vi "rsscope_core_global.vi"() -> ()   [LabVIEW 2014] (continued)
"Access"=2, "Range Table"="RsScope_rngPowerQualityCustomFrequency", "Read Callback"="", "Write Callback"="", "Supported Models"="", "Instrument Options"="", "Flags"=0, "Help"="Sets the user-defined frequency if RSSCOPE_ATTR_POWER_QUALITY_FREQUENCY is set to Custom.\n\nAvailable Repeated Capabilities:\nNone\n\nRemote-control command(s):\nPOWer:QUALity:FCUS"}, {"Level"=3, "Class Only"=FALSE, "Identifier"="RSSCOPE_ATTR_POWER_QUALITY_SCALING", "Descriptive Name"="Power Quality Scaling", "Data Type"=0, "Command"="POW:QUAL:AUTO", "Access"=2, "Range Table"="RsScope_rngPowerScaling", "Read Callback"="", "Write Callback"="", "Supported Models"="", "Instrument Options"="", "Flags"=0, "Help"="Selects the scaling for the display of the results.\n\nAvailable Repeated Capabilities:\nNone\n\nRemote-control command(s):\nPOWer:QUALity:AUTO"}, {"Level"=3, "Class Only"=FALSE, "Identifier"="RSSCOPE_ATTR_POWER_QUALITY_ADD", "Descriptive Name"="Power Quality Add To Report", "Data Type"=4, "Command"="POW:QUAL:REP:ADD", "Access"=1, "Range Table"="", "Read Callback"="", "Write Callback"="", "Supported Models"="", "Instrument Options"="", "Flags"=0, "Help"="Adds the result to the report list.\n\nAvailable Repeated Capabilities:\nNone\n\nRemote-control command(s):\nPOWer:QUALity:REPort:ADD"}, {"Level"=3, "Class Only"=TRUE, "Identifier"="", "Descriptive Name"="Results", "Data Type"=0, "Command"="", "Access"=0, "Range Table"="", "Read Callback"="", "Write Callback"="", "Supported Models"="", "Instrument Options"="", "Flags"=0, "Help"="Power quality measurement results."}, {"Level"=2, "Class Only"=TRUE, "Identifier"="", "Descriptive Name"="Current Harmonics", "Data Type"=0, "Command"="", "Access"=0, "Range Table"="", "Read Callback"="", "Write Callback"="", "Supported Models"="", "Instrument Options"="", "Flags"=0, "Help"="Current Harmonics"}, {"Level"=3, "Class Only"=FALSE, "Identifier"="RSSCOPE_ATTR_START_POWER_CURRENT_HARMONICS", "Descriptive Name"="Start Power Current Harmonics Measurement", "Data Type"=4, "Command"="POW:HARM:EXEC", "Access"=1, "Range Table"="", "Read Callback"="", "Write Callback"="", "Supported Models"="", "Instrument Options"="", "Flags"=0, "Help"="Start power current harmonics measurement.\n\nAvailable Repeated Capabilities:\nNone\n\nRemote-control command(s):\nPOWer:HARMonics:EXECute"}, {"Level"=3, "Class Only"=FALSE, "Identifier"="RSSCOPE_ATTR_POWER_CURRENT_HARMONICS_STANDARD", "Descriptive Name"="Power Current Harmonics Standard", "Data Type"=0, "Command"="POW:HARM:STAN", "Access"=2, "Range Table"="RsScope_rngPowerCurrentHarmonicsStandard", "Read Callback"="", "Write Callback"="", "Supported Models"="", "Instrument Options"="", "Flags"=0, "Help"="Selects current harmonics standard.\n\nAvailable Repeated Capabilities:\nNone\n\nRemote-control command(s):\nPOWer:HARMonics:STAN"}, {"Level"=3, "Class Only"=FALSE, "Identifier"="RSSCOPE_ATTR_POWER_CURRENT_HARMONICS_EN_FREQUENCY", "Descriptive Name"="Power Current Harmonics EN Frequency", "Data Type"=0, "Command"="POW:HARM:ENFR", "Access"=2, "Range Table"="RsScope_rngPowerCurrentHarmonicsFrequency", "Read Callback"="", "Write Callback"="", "Supported Models"="", "Instrument Options"="", "Flags"=0, "Help"="Selects the frequency of the input signal for the EN 61000-3-2 Class standards.\nValues F_50 and F_60 are valid for this command.\n\nAvailable Repeated Capabilities:\nNone\n\nRemote-control command(s):\nPOWer:HARMonics:ENFR"}, {"Level"=3, "Class Only"=FALSE, "Identifier"="RSSCOPE_ATTR_POWER_CURRENT_HARMONICS_MI_FREQUENCY", "Descriptive Name"="Power Current Harmonics MI Frequency", "Data Type"=0, "Command"="POW:HARM:MIFR", "Access"=2, "Range Table"="RsScope_rngPowerCurrentHarmonicsFrequency", "Read Callback"="", "Write Callback"="", "Supported Models"="", "Instrument Options"="", "Flags"=0, "Help"="Selects the frequency of the input signal for the MIL-STD-1399 standard.\nF_60 and F_400 are valid for this command\n\nAvailable Repeated Capabilities:\nNone\n\nRemote-control command(s):\nPOWer:HARMonics:MIFR"}, {"Level"=3, "Class Only"=FALSE, "Identifier"="RSSCOPE_ATTR_POWER_CURRENT_HARMONICS_DO_FREQUENCY", "Descriptive Name"="Power Current Harmonics DO Frequency", "Data Type"=0, "Command"="POW:HARM:DOFR", "Access"=2, "Range Table"="RsScope_rngPowerCurrentHarmonicsFrequency", "Read Callback"="", "Write Callback"="", "Supported Models"="", "Instrument Options"="", "Flags"=0, "Help"="Selects the frequency of the input signal for theRTCA DO-160 standard.\nValues F_360, F_400, F_650, F_800 are valid for this command\n\nAvailable Repeated Capabilities:\nNone\n\nRemote-control command(s):\nPOWer:HARMonics:DOFR"}, {"Level"=3, "Class Only"=FALSE, "Identifier"="RSSCOPE_ATTR_POWER_CURRENT_HARMONICS_EVALUATION", "Descriptive Name"="Power Current Harmonics Evaluation", "Data Type"=0, "Command"="POW:HARM:EVAL", "Access"=2, "Range Table"="RsScope_rngPowerCurrentHarmonicsEvaluation", "Read Callback"="", "Write Callback"="", "Supported Models"="", "Instrument Options"="", "Flags"=0, "Help"="Selects how the results are evaluated.\n\nAvailable Repeated Capabilities:\nNone\n\nRemote-control command(s):\nPOWer:HARMonics:EVAL"}, {"Level"=3, "Class Only"=FALSE, "Identifier"="RSSCOPE_ATTR_POWER_CURRENT_HARMONICS_EVALUATION_VOLT", "Descriptive Name"="Power Current Harmonics Evaluation Voltage", "Data Type"=0, "Command"="POW:HARM:VOLT", "Access"=2, "Range Table"="RsScope_rngPowerCurrentHarmonicsVoltageResultsDisplay", "Read Callback"="", "Write Callback"="", "Supported Models"="", "Instrument Options"="", "Flags"=0, "Help"="Selects if the voltage results are displayed or not for &apos;Standard&apos; > &apos;RTCA DO-160&apos; and enabled &apos;Evaluation with voltage source and revised current law&apos;.\n\nAvailable Repeated Capabilities:\nNone\n\nRemote-control command(s):\nPOWer:HARMonics:VOLT"}, {"Level"=3, "Class Only"=FALSE, "Identifier"="RSSCOPE_ATTR_POWER_CURRENT_HARMONICS_SCALING", "Descriptive Name"="Power Current Harmonics Scaling", "Data Type"=0, "Command"="POW:HARM:AUTO", "Access"=2, "Range Table"="RsScope_rngPowerScaling", "Read Callback"="", "Write Callback"="", "Supported Models"="", "Instrument Options"="", "Flags"=0, "Help"="Selects the scaling for the display of the results.\n\nAvailable Repeated Capabilities:\nNone\n\nRemote-control command(s):\nPOWer:HARMonics:AUTO"}, {"Level"=3, "Class Only"=FALSE, "Identifier"="RSSCOPE_ATTR_POWER_CURRENT_HARMONICS_ADD", "Descriptive Name"="Power Current Harmonics Add To Report", "Data Type"=4, "Command"="POW:HARM:REP:ADD", "Access"=1, "Range Table"="", "Read Callback"="", "Write Callback"="", "Supported Models"="", "Instrument Options"="", "Flags"=0, "Help"="Adds the result to the report list.\n\nAvailable Repeated Capabilities:\nNone\n\nRemote-control command(s):\nPOWer:HARMonics:REPort:ADD"}, {"Level"=3, "Class Only"=TRUE, "Identifier"="", "Descriptive Name"="Results", "Data Type"=0, "Command"="", "Access"=0, "Range Table"="", "Read Callback"="", "Write Callback"="", "Supported Models"="", "Instrument Options"="", "Flags"=0, "Help"="Current harmonics measurement results."}, {"Level"=4, "Class Only"=FALSE, "Identifier"="RSSCOPE_ATTR_POWER_CURRENT_HARMONICS_USED_STANDARD", "Descriptive Name"="Power Current Harmonics Used Standard", "Data Type"=0, "Command"="POW:HARM:RES{ResultNumber}:STD?", "Access"=0, "Range Table"="RsScope_rngPowerCurrentHarmonicsStandard", "Read Callback"="", "Write Callback"="", "Supported Models"="", "Instrument Options"="", "Flags"=0, "Help"="Returns the used standard.\n\nAvailable Repeated Capabilities:\nResultNumber: Res1, Res2, Res3, Res4, Res5, Res6, Res7, Res8\r\n\nRemote-control command(s):\nPOWer:HARMonics:RESult<m>:STDinuse?"}, {"Level"=4, "Class Only"=TRUE, "Identifier"="", "Descriptive Name"="Harmonic", "Data Type"=0, "Command"="", "Access"=0, "Range Table"="", "Read Callback"="", "Write Callback"="", "Supported Models"="", "Instrument Options"="", "Flags"=0, "Help"="Functions with repeated capabilty ResultHarmonics"}, {"Level"=5, "Class Only"=FALSE, "Identifier"="RSSCOPE_ATTR_POWER_CURRENT_HARMONICS_RESULT_FREQUENCY", "Descriptive Name"="Power Current Harmonics Result Frequency", "Data Type"=1, "Command"="POW:HARM:RES{ResultNumber}:FREQ{ResultHarmonics}:VAL?", "Access"=0, "Range Table"="", "Read Callback"="", "Write Callback"="", "Supported Models"="", "Instrument Options"="", "Flags"=0, "Help"="Returns the frequency for selected result and harmonic.\n\nAvailable Repeated Capabilities:\nResultNumber: Res1, Res2, Res3, Res4, Res5, Res6, Res7, Res8\r\nResultHarmonics: Harm1, Harm2, Harm3, Harm4, Harm5, Harm6, Harm7, Harm8, Harm9, Harm10, Harm11, Harm12, Harm13, Harm14, Harm15, Harm16, Harm17, Harm18, Harm19, Harm20, Harm21, Harm22, Harm23, Harm24, Harm25, Harm26, Harm27, Harm28, Harm29, Harm30, Harm31, Harm32, Harm33, Harm34, Harm35, Harm36, Harm37, Harm38, Harm39, Herm40\r\n\nRemote-control command(s):\nPOWer:HARMonics:RESult<m>:FREQuency<n>:VALue?"}, {"Level"=5, "Class Only"=FALSE, "Identifier"="RSSCOPE_ATTR_POWER_CURRENT_HARMONICS_RESULT_MAX", "Descriptive Name"="Power Current Harmonics Result Maximum", "Data Type"=1, "Command"="POW:HARM:RES{ResultNumber}:MAXV{ResultHarmonics}:VAL?", "Access"=0, "Range Table"="", "Read Callback"="", "Write Callback"="", "Supported Models"="", "Instrument Options"="", "Flags"=0, "Help"="Returns the maximum measured value for selected result and harmonic.\n\nAvailable Repeated Capabilities:\nResultNumber: Res1, Res2, Res3, Res4, Res5, Res6, Res7, Res8\r\nResultHarmonics: Harm1, Harm2, Harm3, Harm4, Harm5, Harm6, Harm7, Harm8, Harm9, Harm10, Harm11, Harm12, Harm13, Harm14, Harm15, Harm16, Harm17, Harm18, Harm19, Harm20, Harm21, Harm22, Harm23, Harm24, Harm25, Harm26, Harm27, Harm28, Harm29, Harm30, Harm31, Harm32, Harm33, Harm34, Harm35, Harm36, Harm37, Harm38, Harm39, Herm40\r\n\nRemote-control command(s):\nPOWer:HARMonics:RESult<m>:MAXValue<n>:VALue?"}, {"Level"=5, "Class Only"=FALSE, "Identifier"="RSSCOPE_ATTR_POWER_CURRENT_HARMONICS_RESULT_STD", "Descriptive Name"="Power Current Harmonics Result Standard Limit", "Data Type"=1, "Command"="POW:HARM:RES{ResultNumber}:STDV{ResultHarmonics}:VAL?", "Access"=0, "Range Table"="", "Read Callback"="", "Write Callback"="", "Supported Models"="", "Instrument Options"="", "Flags"=0, "Help"="Returns the maxim alowed value according selected standard for selected result and harmonic.\n\nAvailable Repeated Capabilities:\nResultNumber: Res1, Res2, Res3, Res4, Res5, Res6, Res7, Res8\r\nResultHarmonics: Harm1, Harm2, Harm3, Harm4, Harm5, Harm6, Harm7, Harm8, Harm9, Harm10, Harm11, Harm12, Harm13, Harm14, Harm15, Harm16, Harm17, Harm18, Harm19, Harm20, Harm21, Harm22, Harm23, Harm24, Harm25, Harm26, Harm27, Harm28, Harm29, Harm30, Harm31, Harm32, Harm33, Harm34, Harm35, Harm36, Harm37, Harm38, Harm39, Herm40\r\n\nRemote-control command(s):\nPOWer:HARMonics:RESult<m>:STDValue<n>:VALue?"}, {"Level"=5, "Class Only"=FALSE, "Identifier"="RSSCOPE_ATTR_POWER_CURRENT_HARMONICS_RESULT_VALUE", "Descriptive Name"="Power Current Harmonics Result Value", "Data Type"=1, "Command"="POW:HARM:RES{ResultNumber}:VAL{ResultHarmonics}:VAL?", "Access"=0, "Range Table"="", "Read Callback"="", "Write Callback"="", "Supported Models"="", "Instrument Options"="", "Flags"=0, "Help"="Returns the present value for selected result and harmonic.\n\nAvailable Repeated Capabilities:\nResultNumber: Res1, Res2, Res3, Res4, Res5, Res6, Res7, Res8\r\nResultHarmonics: Harm1, Harm2, Harm3, Harm4, Harm5, Harm6, Harm7, Harm8, Harm9, Harm10, Harm11, Harm12, Harm13, Harm14, Harm15, Harm16, Harm17, Harm18, Harm19, Harm20, Harm21, Harm22, Harm23, Harm24, Harm25, Harm26, Harm27, Harm28, Harm29, Harm30, Harm31, Harm32, Harm33, Harm34, Harm35, Harm36, Harm37, Harm38, Harm39, Herm40\r\n\nRemote-control command(s):\nPOWer:HARMonics:RESult<m>:VALue<n>:VALue?"}, {"Level"=2, "Class Only"=TRUE, "Identifier"="", "Descriptive Name"="Inrush Current", "Data Type"=0, "Command"="", "Access"=0, "Range Table"="", "Read Callback"="", "Write Callback"="", "Supported Models"="", "Instrument Options"="", "Flags"=0, "Help"="Inrush current measurement."}, {"Level"=3, "Class Only"=FALSE, "Identifier"="RSSCOPE_ATTR_START_POWER_INRUSH_CURRENT_MEASUREMENT", "Descriptive Name"="Start Power Inrush Current Measurement", "Data Type"=4, "Command"="POW:INR:EXEC", "Access"=1, "Range Table"="", "Read Callback"="", "Write Callback"="", "Supported Models"="", "Instrument Options"="", "Flags"=0, "Help"="Start power inrush current measurement.\n\nAvailable Repeated Capabilities:\nNone\n\nRemote-control command(s):\nPOWer:INRush:EXECute"}, {"Level"=3, "Class Only"=FALSE, "Identifier"="RSSCOPE_ATTR_POWER_INRUSH_CURRENT_MAX", "Descriptive Name"="Power Inrush Current Max Current", "Data Type"=1, "Command"="POW:INR:MAXC", "Access"=2, "Range Table"="RsScope_rngPowerInrushCurrentMaxCurrent", "Read Callback"="", "Write Callback"="", "Supported Models"="", "Instrument Options"="", "Flags"=0, "Help"="Sets the maximum expected current for the vertical scale.\n\nAvailable Repeated Capabilities:\nNone\n\nRemote-control command(s):\nPOWer:INRush:MAXCurrent"}, {"Level"=3, "Class Only"=FALSE, "Identifier"="RSSCOPE_ATTR_POWER_INRUSH_CURRENT_TRIGGER", "Descriptive Name"="Power Inrush Current Trigger", "Data Type"=1, "Command"="POW:INR:TRIG", "Access"=2, "Range Table"="RsScope_rngPowerInrushCurrentTrigger", "Read Callback"="", "Write Callback"="", "Supported Models"="", "Instrument Options"="", "Flags"=0, "Help"="Sets the current value for the trigger\n\nAvailable Repeated Capabilities:\nNone\n\nRemote-control command(s):\nPOWer:INRush:TRIGger"}, {"Level"=3, "Class Only"=FALSE, "Identifier"="RSSCOPE_ATTR_POWER_INRUSH_CURRENT_ADD", "Descriptive Name"="Power Inrush Current Add To Report", "Data Type"=4, "Command"="POW:INR:REP:ADD", "Access"=1, "Range Table"="", "Read Callback"="", "Write Callback"="", "Supported Models"="", "Instrument Options"="", "Flags"=0, "Help"="Adds the result to the report list.\n\nAvailable Repeated Capabilities:\nNone\n\nRemote-control command(s):\nPOWer:INRush:REPort:ADD"}, {"Level"=3, "Class Only"=FALSE, "Identifier"="RSSCOPE_ATTR_POWER_INRUSH_CURRENT_GATE_ADD", "Descriptive Name"="Power Inrush Current Gate Add", "Data Type"=4, "Command"="POW:INR:ADD", "Access"=1, "Range Table"="", "Read Callback"="", "Write Callback"="", "Supported Models"="", "Instrument Options"="", "Flags"=0, "Help"="Adds a gate.\n\nAvailable Repeated Capabilities:\nNone\n\nRemote-control command(s):\nPOWer:INRush:ADD"}, {"Level"=3, "Class Only"=FALSE, "Identifier"="RSSCOPE_ATTR_POWER_INRUSH_CURRENT_GATE_INS", "Descriptive Name"="Power Inrush Current Gate Insert", "Data Type"=0, "Command"="POW:INR:INS", "Access"=1, "Range Table"="", "Read Callback"="", "Write Callback"="", "Supported Models"="", "Instrument Options"="", "Flags"=0, "Help"="Inserts a gate.\n\nAvailable Repeated Capabilities:\nNone\n\nRemote-control command(s):\nPOWer:INRush:INSert"}, {"Level"=3, "Class Only"=FALSE, "Identifier"="RSSCOPE_ATTR_POWER_INRUSH_CURRENT_GATE_REMOVE", "Descriptive Name"="Power Inrush Current Gate Remove", "Data Type"=0, "Command"="POW:INR:REM", "Access"=1, "Range Table"="", "Read Callback"="", "Write Callback"="", "Supported Models"="", "Instrument Options"="", "Flags"=0, "Help"="Removes a gate.\n\nAvailable Repeated Capabilities:\nNone\n\nRemote-control command(s):\nPOWer:INRush:REMove"}, {"Level"=3, "Class Only"=FALSE, "Identifier"="RSSCOPE_ATTR_POWER_INRUSH_CURRENT_GATE_COUNT", "Descriptive Name"="Power Inrush Current Gate Count", "Data Type"=0, "Command"="POW:INR:COUN?", "Access"=0, "Range Table"="", "Read Callback"="", "Write Callback"="", "Supported Models"="", "Instrument Options"="", "Flags"=0, "Help"="Queiries the number of inrush current gates.\n\nAvailable Repeated Capabilities:\nNone\n\nRemote-control command(s):\nPOWer:INRush:COUNt?"}, {"Level"=3, "Class Only"=TRUE, "Identifier"="", "Descriptive Name"="Gate", "Data Type"=0, "Command"="", "Access"=0, "Range Table"="", "Read Callback"="", "Write Callback"="", "Supported Models"="", "Instrument Options"="", "Flags"=0, "Help"="Attributes with gate repeated capability.\n\nConfigures different gates (time periods). You can configure up to\nfive different gates. The time periods of the defined gates may overlap."}, {"Level"=4, "Class Only"=FALSE, "Identifier"="RSSCOPE_ATTR_POWER_INRUSH_CURRENT_GATE_VALUE", "Descriptive Name"="Power Inrush Current Gate Value", "Data Type"=1, "Command"="POW:INR:GATE{Gate}:VAL", "Access"=2, "Range Table"="RsScope_rngPowerInrushCurrentGateValue", "Read Callback"="", "Write Callback"="", "Supported Models"="", "Instrument Options"="", "Flags"=0, "Help"="Sets the value of the inrush current.\n\nAvailable Repeated Capabilities:\nGate: Gate1, Gate2, Gate3, Gate4, Gate5\r\n\nRemote-control command(s):\nPOWer:INRush:GATE<m>:VAlue"}, {"Level"=4, "Class Only"=FALSE, "Identifier"="RSSCOPE_ATTR_POWER_INRUSH_CURRENT_GATE_START", "Descriptive Name"="Power Inrush Current Gate Start", "Data Type"=1, "Command"="POW:INR:GATE{Gate}:STAR", "Access"=2, "Range Table"="RsScope_rngPowerInrushCurrentGateMeasTime", "Read Callback"="", "Write Callback"="", "Supported Models"="", "Instrument Options"="", "Flags"=0, "Help"="Sets the start measuring time for the selected gate.\n\nAvailable Repeated Capabilities:\nGate: Gate1, Gate2, Gate3, Gate4, Gate5\r\n\nRemote-control command(s):\nPOWer:INRush:GATE<m>:STARt"}, {"Level"=4, "Class Only"=FALSE, "Identifier"="RSSCOPE_ATTR_POWER_INRUSH_CURRENT_GATE_STOP", "Descriptive Name"="Power Inrush Current Gate Stop", "Data Type"=1, "Command"="POW:INR:GATE{Gate}:STOP", "Access"=2, "Range Table"="RsScope_rngPowerInrushCurrentGateMeasTime", "Read Callback"="", "Write Callback"="", "Supported Models"="", "Instrument Options"="", "Flags"=0, "Help"="Sets the stop measuring time for the selected gate.\n\nAvailable Repeated Capabilities:\nGate: Gate1, Gate2, Gate3, Gate4, Gate5\r\n\nRemote-control command(s):\nPOWer:INRush:GATE<m>:STOP"}, {"Level"=4, "Class Only"=FALSE, "Identifier"="RSSCOPE_ATTR_POWER_INRUSH_CURRENT_RESULT_VALUE", "Descriptive Name"="Power Inrush Current Result Value", "Data Type"=1, "Command"="POW:INR:GATE{Gate}:VAL?", "Access"=0, "Range Table"="", "Read Callback"="", "Write Callback"="", "Supported Models"="", "Instrument Options"="", "Flags"=0, "Help"="Returns the value of the inrush current.\n\nAvailable Repeated Capabilities:\nGate: Gate1, Gate2, Gate3, Gate4, Gate5\r\n\nRemote-control command(s):\nPOWer:INRush:GATE<m>:VALue?"}, {"Level"=2, "Class Only"=TRUE, "Identifier"="", "Descriptive Name"="Ripple", "Data Type"=0, "Command"="", "Access"=0, "Range Table"="", "Read Callback"="", "Write Callback"="", "Supported Models"="", "Instrument Options"="", "Flags"=0, "Help"="Measures the ripple of the device output."}, {"Level"=3, "Class Only"=FALSE, "Identifier"="RSSCOPE_ATTR_START_POWER_RIPPLE_MEASUREMENT", "Descriptive Name"="Start Power Ripple Measurement", "Data Type"=4, "Command"="POW:RIPP:EXEC", "Access"=1, "Range Table"="", "Read Callback"="", "Write Callback"="", "Supported Models"="", "Instrument Options"="", "Flags"=0, "Help"="Start power ripple measurement.\n\nAvailable Repeated Capabilities:\nNone\n\nRemote-control command(s):\nPOWer:RIPPle:EXECute"}, {"Level"=3, "Class Only"=FALSE, "Identifier"="RSSCOPE_ATTR_POWER_RIPPLE_CURRENT_ENABLED", "Descriptive Name"="Power Ripple Current Enabled", "Data Type"=3, "Command"="POW:RIPP:CURR", "Access"=2, "Range Table"="", "Read Callback"="", "Write Callback"="", "Supported Models"="", "Instrument Options"="", "Flags"=0, "Help"="Activates or deactivates the input current.\n\nAvailable Repeated Capabilities:\nNone\n\nRemote-control command(s):\nPOWer:RIPPle:CURRent"}, {"Level"=3, "Class Only"=FALSE, "Identifier"="RSSCOPE_ATTR_POWER_RIPPLE_FREQUENCY", "Descriptive Name"="Power Ripple Frequency", "Data Type"=1, "Command"="POW:RIPP:FREQ", "Access"=2, "Range Table"="RsScope_rngPowerSwitchingFrequency", "Read Callback"="", "Write Callback"="", "Supported Models"="", "Instrument Options"="", "Flags"=0, "Help"="Sets the SMPS switching frequency.\n\nAvailable Repeated Capabilities:\nNone\n\nRemote-control command(s):\nPOWer:RIPPle:FREQuency"}, {"Level"=3, "Class Only"=FALSE, "Identifier"="RSSCOPE_ATTR_POWER_RIPPLE_SCALING", "Descriptive Name"="Power Ripple Scaling", "Data Type"=0, "Command"="POW:RIPP:AUT", "Access"=2, "Range Table"="RsScope_rngPowerScaling", "Read Callback"="", "Write Callback"="", "Supported Models"="", "Instrument Options"="", "Flags"=0, "Help"="Selects the scaling for the display of the results.\n\nAvailable Repeated Capabilities:\nNone\n\nRemote-control command(s):\nPOWer:RIPPle:AUToscale"}, {"Level"=3, "Class Only"=FALSE, "Identifier"="RSSCOPE_ATTR_POWER_RIPPLE_ADD", "Descriptive Name"="Power Ripple Add To Report", "Data Type"=4, "Command"="POW:RIPP:REP:ADD", "Access"=1, "Range Table"="", "Read Callback"="", "Write Callback"="", "Supported Models"="", "Instrument Options"="", "Flags"=0, "Help"="Adds the result to the report list.\n\nAvailable Repeated Capabilities:\nNone\n\nRemote-control command(s):\nPOWer:RIPPle:REPort:ADD"}, {"Level"=3, "Class Only"=TRUE, "Identifier"="", "Descriptive Name"="Results", "Data Type"=0, "Command"="", "Access"=0, "Range Table"="", "Read Callback"="", "Write Callback"="", "Supported Models"="", "Instrument Options"="", "Flags"=0, "Help"="Results of the ripple analysis."}, {"Level"=2, "Class Only"=TRUE, "Identifier"="", "Descriptive Name"="Spectrum", "Data Type"=0, "Command"="", "Access"=0, "Range Table"="", "Read Callback"="", "Write Callback"="", "Supported Models"="", "Instrument Options"="", "Flags"=0, "Help"="Power spectrum measurement."}, {"Level"=3, "Class Only"=FALSE, "Identifier"="RSSCOPE_ATTR_START_POWER_SPECTRUM_MEASUREMENT", "Descriptive Name"="Start Power Spectrum Measurement", "Data Type"=4, "Command"="POW:SPEC:EXEC", "Access"=1, "Range Table"="", "Read Callback"="", "Write Callback"="", "Supported Models"="", "Instrument Options"="", "Flags"=0, "Help"="Starts the spectrum measurement.\n\nAvailable Repeated Capabilities:\nNone\n\nRemote-control command(s):\nPOWer:SPECtrum:EXECute"}, {"Level"=3, "Class Only"=FALSE, "Identifier"="RSSCOPE_ATTR_POWER_SPECTRUM_FREQUENCY", "Descriptive Name"="Power Spectrum Frequency", "Data Type"=1, "Command"="POW:SPEC:FREQ", "Access"=2, "Range Table"="RsScope_rngPowerSwitchingFrequency", "Read Callback"="", "Write Callback"="", "Supported Models"="", "Instrument Options"="", "Flags"=0, "Help"="Sets the SMPS switching frequency.\n\nAvailable Repeated Capabilities:\nNone\n\nRemote-control command(s):\nPOWer:SPECtrum:FREQuency"}, {"Level"=3, "Class Only"=FALSE, "Identifier"="RSSCOPE_ATTR_POWER_SPECTRUM_SCALING", "Descriptive Name"="Power Spectrum Scaling", "Data Type"=0, "Command"="POW:SPEC:AUT", "Access"=2, "Range Table"="RsScope_rngPowerScaling", "Read Callback"="", "Write Callback"="", "Supported Models"="", "Instrument Options"="", "Flags"=0, "Help"="Selects the scaling for the display of the results.\n\nAvailable Repeated Capabilities:\nNone\n\nRemote-control command(s):\nPOWer:SPECtrum:AUToscale"}, {"Level"=3, "Class Only"=FALSE, "Identifier"="RSSCOPE_ATTR_POWER_SPECTRUM_ADD", "Descriptive Name"="Power Spectrum Add To Report", "Data Type"=4, "Command"="POW:SPEC:REP:ADD", "Access"=1, "Range Table"="", "Read Callback"="", "Write Callback"="", "Supported Models"="", "Instrument Options"="", "Flags"=0, "Help"="Adds the result to the report list.\n\nAvailable Repeated Capabilities:\nNone\n\nRemote-control command(s):\nPOWer:SPECtrum:REPort:ADD"}, {"Level"=3, "Class Only"=TRUE, "Identifier"="", "Descriptive Name"="Results", "Data Type"=0, "Command"="", "Access"=0, "Range Table"="", "Read Callback"="", "Write Callback"="", "Supported Models"="", "Instrument Options"="", "Flags"=0, "Help"="Power Spectrum Measurement Results."}, {"Level"=4, "Class Only"=FALSE, "Identifier"="RSSCOPE_ATTR_POWER_SPECTRUM_MEASUREMENT_RESULT_COUNT", "Descriptive Name"="Result Count", "Data Type"=0, "Command"="POW:SPEC:RCO?", "Access"=0, "Range Table"="", "Read Callback"="", "Write Callback"="", "Supported Models"="", "Instrument Options"="", "Flags"=0, "Help"="Returns the total number of harmonics.\n\nAvailable Repeated Capabilities:\nNone\n\nRemote-control command(s):\nPOWer:SPECtrum:RCOunt?"}, {"Level"=4, "Class Only"=FALSE, "Identifier"="RSSCOPE_ATTR_POWER_SPECTRUM_MEASUREMENT_FREQUENCY_RESULT", "Descriptive Name"="Power Spectrum Measurement Frequency Result", "Data Type"=1, "Command"="POW:SPEC:RES{ResultNumber}:FREQ?", "Access"=0, "Range Table"="", "Read Callback"="", "Write Callback"="", "Supported Models"="", "Instrument Options"="", "Flags"=0, "Help"="Returns the result frequency.\n\nAvailable Repeated Capabilities:\nResultNumber: Res1, Res2, Res3, Res4, Res5, Res6, Res7, Res8\r\n\nRemote-control command(s):\nPOWer:SPECtrum:RESult<m>:FREQuency?"}, {"Level"=4, "Class Only"=FALSE, "Identifier"="RSSCOPE_ATTR_POWER_SPECTRUM_MEASUREMENT_LEVEL_RESULT", "Descriptive Name"="Power Spectrum Measurement Level Result", "Data Type"=1, "Command"="POW:SPEC:RES{ResultNumber}:LEV?", "Access"=0, "Range Table"="", "Read Callback"="", "Write Callback"="", "Supported Models"="", "Instrument Options"="", "Flags"=0, "Help"="Returns the result level.\n\nAvailable Repeated Capabilities:\nResultNumber: Res1, Res2, Res3, Res4, Res5, Res6, Res7, Res8\r\n\nRemote-control command(s):\nPOWer:SPECtrum:RESult<m>:LEVel?"}, {"Level"=2, "Class Only"=TRUE, "Identifier"="", "Descriptive Name"="Slew Rate", "Data Type"=0, "Command"="", "Access"=0, "Range Table"="", "Read Callback"="", "Write Callback"="", "Supported Models"="", "Instrument Options"="", "Flags"=0, "Help"="Slew rate measurement."}, {"Level"=3, "Class Only"=FALSE, "Identifier"="RSSCOPE_ATTR_START_POWER_SLEW_RATE_MEASUREMENT", "Descriptive Name"="Start Power Slew Rate Measurement", "Data Type"=4, "Command"="POW:SLEW:EXEC", "Access"=1, "Range Table"="", "Read Callback"="", "Write Callback"="", "Supported Models"="", "Instrument Options"="", "Flags"=0, "Help"="Starts the slew rate measurement.\n\nAvailable Repeated Capabilities:\nNone\n\nRemote-control command(s):\nPOWer:SLEWrate:EXECute"}, {"Level"=3, "Class Only"=FALSE, "Identifier"="RSSCOPE_ATTR_POWER_SLEW_RATE_SOURCE", "Descriptive Name"="Power Slew Rate Source", "Data Type"=0, "Command"="POW:SLEW:SOUR", "Access"=2, "Range Table"="RsScope_rngPowerSource", "Read Callback"="", "Write Callback"="", "Supported Models"="", "Instrument Options"="", "Flags"=0, "Help"="Selects the source for the measurement.\n\nAvailable Repeated Capabilities:\nNone\n\nRemote-control command(s):\nPOWer:SLEWrate:SOURce"}, {"Level"=3, "Class Only"=FALSE, "Identifier"="RSSCOPE_ATTR_POWER_SLEW_RATE_AVERAGE", "Descriptive Name"="Power Slew Rate Average", "Data Type"=3, "Command"="POW:SLEW:AVGD", "Access"=2, "Range Table"="", "Read Callback"="", "Write Callback"="", "Supported Models"="", "Instrument Options"="", "Flags"=0, "Help"="Enables/disables averaging.\n\nAvailable Repeated Capabilities:\nNone\n\nRemote-control command(s):\nPOWer:SLEWrate:AVGDeriv"}, {"Level"=3, "Class Only"=FALSE, "Identifier"="RSSCOPE_ATTR_POWER_SLEW_RATE_SCALING", "Descriptive Name"="Power Slew Rate Scaling", "Data Type"=0, "Command"="POW:SLEW:AUTO", "Access"=2, "Range Table"="RsScope_rngPowerScaling", "Read Callback"="", "Write Callback"="", "Supported Models"="", "Instrument Options"="", "Flags"=0, "Help"="Selects the scaling for the display of the results.\n\nAvailable Repeated Capabilities:\nNone\n\nRemote-control command(s):\nPOWer:SLEWrate:AUTO"}, {"Level"=3, "Class Only"=FALSE, "Identifier"="RSSCOPE_ATTR_POWER_SLEW_RATE_ADD", "Descriptive Name"="Power Slew Rate Add To Report", "Data Type"=4, "Command"="POW:SLEW:REP:ADD", "Access"=1, "Range Table"="", "Read Callback"="", "Write Callback"="", "Supported Models"="", "Instrument Options"="", "Flags"=0, "Help"="Adds the result to the report list.\n\nAvailable Repeated Capabilities:\nNone\n\nRemote-control command(s):\nPOWer:SLEWrate:REPort:ADD"}, {"Level"=3, "Class Only"=TRUE, "Identifier"="", "Descriptive Name"="Gate", "Data Type"=0, "Command"="", "Access"=0, "Range Table"="", "Read Callback"="", "Write Callback"="", "Supported Models"="", "Instrument Options"="", "Flags"=0, "Help"="Attributes with gate repeated capability."}, {"Level"=4, "Class Only"=FALSE, "Identifier"="RSSCOPE_ATTR_POWER_SLEW_RATE_GATE_START", "Descriptive Name"="Power Slew Rate Gate Start", "Data Type"=1, "Command"="POW:SLEW:GATE:STARt", "Access"=2, "Range Table"="", "Read Callback"="", "Write Callback"="", "Supported Models"="", "Instrument Options"="", "Flags"=0, "Help"="Start of the gate.\n\nAvailable Repeated Capabilities:\nNone\n\nRemote-control command(s):\nPOWer:SLEWrate:GATE:STARt"}, {"Level"=4, "Class Only"=FALSE, "Identifier"="RSSCOPE_ATTR_POWER_SLEW_RATE_GATE_STOP", "Descriptive Name"="Power Slew Rate Gate Stop", "Data Type"=1, "Command"="POW:SLEWrate:GATE:STOP", "Access"=2, "Range Table"="", "Read Callback"="", "Write Callback"="", "Supported Models"="", "Instrument Options"="", "Flags"=0, "Help"="Stop of the gate.\n\nAvailable Repeated Capabilities:\nNone\n\nRemote-control command(s):\nPOWer:SLEWrate:GATE:STOP"}, {"Level"=3, "Class Only"=TRUE, "Identifier"="", "Descriptive Name"="Results", "Data Type"=0, "Command"="", "Access"=0, "Range Table"="", "Read Callback"="", "Write Callback"="", "Supported Models"="", "Instrument Options"="", "Flags"=0, "Help"="Slew rate measurement results."}, {"Level"=2, "Class Only"=TRUE, "Identifier"="", "Descriptive Name"="Safe Operating Area", "Data Type"=0, "Command"="", "Access"=0, "Range Table"="", "Read Callback"="", "Write Callback"="", "Supported Models"="", "Instrument Options"="", "Flags"=0, "Help"="Configures the Safe Operating Area.\nThe safe operating area is defined by the voltage and current conditions over which a\npower semiconductor device is expected to operate without self-damage. The &apos;Safe\nOperating Area&apos; analysis provides a diagram of the safe operating conditions of your\ndevice."}, {"Level"=3, "Class Only"=FALSE, "Identifier"="RSSCOPE_ATTR_START_POWER_SAFE_OPERATING_AREA_MEASUREMENT", "Descriptive Name"="Start Power Safe Operating Area Measurement", "Data Type"=4, "Command"="POW:SOA:EXEC", "Access"=1, "Range Table"="", "Read Callback"="", "Write Callback"="", "Supported Models"="", "Instrument Options"="", "Flags"=0, "Help"="Starts the safe operating area measurement.\n\nAvailable Repeated Capabilities:\nNone\n\nRemote-control command(s):\nPOWer:SOA:EXECute"}, {"Level"=3, "Class Only"=FALSE, "Identifier"="RSSCOPE_ATTR_SAFE_OPERATING_AREA_MASK_TEST", "Descriptive Name"="Safe Operating Area Mask Test", "Data Type"=3, "Command"="POW:SOA:MASK", "Access"=2, "Range Table"="", "Read Callback"="", "Write Callback"="", "Supported Models"="", "Instrument Options"="", "Flags"=0, "Help"="Activates or deactivates a mask.\n\nAvailable Repeated Capabilities:\nNone\n\nRemote-control command(s):\nPOWer:SOA:MASK"}, {"Level"=3, "Class Only"=FALSE, "Identifier"="RSSCOPE_ATTR_SAFE_OPERATING_AREA_SCALE", "Descriptive Name"="Safe Operating Area Scale", "Data Type"=0, "Command"="POW:SOA:SCAL", "Access"=2, "Range Table"="RsScope_rngPowerSafeOperatingAreaScale", "Read Callback"="", "Write Callback"="", "Supported Models"="", "Instrument Options"="", "Flags"=0, "Help"="Sets the scale for the measurement.\n\nAvailable Repeated Capabilities:\nNone\n\nRemote-control command(s):\nPOWer:SOA:SCALe"}, {"Level"=3, "Class Only"=FALSE, "Identifier"="RSSCOPE_ATTR_SAFE_OPERATING_AREA_SWITCH", "Descriptive Name"="Safe Operating Area Switch", "Data Type"=0, "Command"="POW:SOA:SWIT", "Access"=2, "Range Table"="RsScope_rngPowerSafeOperatingAreaSwitch", "Read Callback"="", "Write Callback"="", "Supported Models"="", "Instrument Options"="", "Flags"=0, "Help"="Switches between linear and logarithmic scale.\n\nAvailable Repeated Capabilities:\nNone\n\nRemote-control command(s):\nPOWer:SOA:SWITch"}, {"Level"=3, "Class Only"=FALSE, "Identifier"="RSSCOPE_ATTR_SAFE_OPERATING_AREA_LIN_ADD", "Descriptive Name"="Safe Operating Area Linear Add", "Data Type"=4, "Command"="POW:SOA:LIN:ADD", "Access"=1, "Range Table"="", "Read Callback"="", "Write Callback"="", "Supported Models"="", "Instrument Options"="", "Flags"=0, "Help"="Adds a point.\n\nAvailable Repeated Capabilities:\nNone\n\nRemote-control command(s):\nPOWer:SOA:LINear:ADD"}, {"Level"=3, "Class Only"=FALSE, "Identifier"="RSSCOPE_ATTR_SAFE_OPERATING_AREA_LIN_INS", "Descriptive Name"="Safe Operating Area Linear Insert", "Data Type"=0, "Command"="POW:SOA:LIN:INS", "Access"=1, "Range Table"="", "Read Callback"="", "Write Callback"="", "Supported Models"="", "Instrument Options"="", "Flags"=0, "Help"="Inserts a point.\n\nAvailable Repeated Capabilities:\nNone\n\nRemote-control command(s):\nPOWer:SOA:LINear:INSert"}, {"Level"=3, "Class Only"=FALSE, "Identifier"="RSSCOPE_ATTR_SAFE_OPERATING_AREA_LIN_REMOVE", "Descriptive Name"="Safe Operating Area Linear Remove", "Data Type"=0, "Command"="POW:SOA:LIN:REM", "Access"=1, "Range Table"="", "Read Callback"="", "Write Callback"="", "Supported Models"="", "Instrument Options"="", "Flags"=0, "Help"="Removes a point.\n\nAvailable Repeated Capabilities:\nNone\n\nRemote-control command(s):\nPOWer:SOA:LINear:REMove"}, {"Level"=3, "Class Only"=FALSE, "Identifier"="RSSCOPE_ATTR_SAFE_OPERATING_AREA_LIN_COUNT", "Descriptive Name"="Safe Operating Area Linear Count", "Data Type"=0, "Command"="POW:SOA:LIN:COUN?", "Access"=0, "Range Table"="", "Read Callback"="", "Write Callback"="", "Supported Models"="", "Instrument Options"="", "Flags"=0, "Help"="Queries the number of points.\n\nAvailable Repeated Capabilities:\nNone\n\nRemote-control command(s):\nPOWer:SOA:LINear:COUNt?"}, {"Level"=3, "Class Only"=FALSE, "Identifier"="RSSCOPE_ATTR_SAFE_OPERATING_AREA_LOG_ADD", "Descriptive Name"="Safe Operating Area Logarithmic Add", "Data Type"=4, "Command"="POW:SOA:LOG:ADD", "Access"=1, "Range Table"="", "Read Callback"="", "Write Callback"="", "Supported Models"="", "Instrument Options"="", "Flags"=0, "Help"="Adds a point.\n\nAvailable Repeated Capabilities:\nNone\n\nRemote-control command(s):\nPOWer:SOA:LOGarithmic:ADD"}, {"Level"=3, "Class Only"=FALSE, "Identifier"="RSSCOPE_ATTR_SAFE_OPERATING_AREA_LOG_INS", "Descriptive Name"="Safe Operating Area Logarithmic Insert", "Data Type"=0, "Command"="POW:SOA:LOG:INS", "Access"=1, "Range Table"="", "Read Callback"="", "Write Callback"="", "Supported Models"="", "Instrument Options"="", "Flags"=0, "Help"="Inserts a point.\n\nAvailable Repeated Capabilities:\nNone\n\nRemote-control command(s):\nPOWer:SOA:LOGarithmic:INSert"}, {"Level"=3, "Class Only"=FALSE, "Identifier"="RSSCOPE_ATTR_SAFE_OPERATING_AREA_LOG_REMOVE", "Descriptive Name"="Safe Operating Area Logarithmic Remove", "Data Type"=0, "Command"="POW:SOA:LOG:REM", "Access"=1, "Range Table"="", "Read Callback"="", "Write Callback"="", "Supported Models"="", "Instrument Options"="", "Flags"=0, "Help"="Removes a point.\n\nAvailable Repeated Capabilities:\nNone\n\nRemote-control command(s):\nPOWer:SOA:LOGarithmic:REMove"}, {"Level"=3, "Class Only"=FALSE, "Identifier"="RSSCOPE_ATTR_SAFE_OPERATING_AREA_LOG_COUNT", "Descriptive Name"="Safe Operating Area Logarithmic Count", "Data Type"=0, "Command"="POW:SOA:LOG:COUN?", "Access"=0, "Range Table"="", "Read Callback"="", "Write Callback"="", "Supported Models"="", "Instrument Options"="", "Flags"=0, "Help"="Queries the number of points.\n\nAvailable Repeated Capabilities:\nNone\n\nRemote-control command(s):\nPOWer:SOA:LOGarithmic:COUNt?"}, {"Level"=3, "Class Only"=FALSE, "Identifier"="RSSCOPE_ATTR_POWER_SAFE_OPERATING_AREA_ADD", "Descriptive Name"="Safe Operating Area Add To Report", "Data Type"=4, "Command"="POW:SOA:REP:ADD", "Access"=1, "Range Table"="", "Read Callback"="", "Write Callback"="", "Supported Models"="", "Instrument Options"="", "Flags"=0, "Help"="Adds the result to the report list.\n\nAvailable Repeated Capabilities:\nNone\n\nRemote-control command(s):\nPOWer:SOA:REPort:ADD"}, {"Level"=2, "Class Only"=TRUE, "Identifier"="", "Descriptive Name"="Modulation Measurement", "Data Type"=0, "Command"="", "Access"=0, "Range Table"="", "Read Callback"="", "Write Callback"="", "Supported Models"="", "Instrument Options"="", "Flags"=0, "Help"="Power modulation measurement."}, {"Level"=3, "Class Only"=FALSE, "Identifier"="RSSCOPE_ATTR_START_POWER_MODULATION_MEASUREMENT", "Descriptive Name"="Start Power Modulation Measurement", "Data Type"=4, "Command"="POW:MOD:EXEC", "Access"=1, "Range Table"="", "Read Callback"="", "Write Callback"="", "Supported Models"="", "Instrument Options"="", "Flags"=0, "Help"="Starts the measurement.\n\nAvailable Repeated Capabilities:\nNone\n\nRemote-control command(s):\nPOWer:MODulation:EXECute"}, {"Level"=3, "Class Only"=FALSE, "Identifier"="RSSCOPE_ATTR_POWER_MODULATION_TYPE", "Descriptive Name"="Power Modulation Type", "Data Type"=0, "Command"="POW:MOD:TYPE", "Access"=2, "Range Table"="RsScope_rngPowerModulationType", "Read Callback"="", "Write Callback"="", "Supported Models"="", "Instrument Options"="", "Flags"=0, "Help"="Selects the type of signal flow for the measurement\n\nAvailable Repeated Capabilities:\nNone\n\nRemote-control command(s):\nPOWer:MODulation:TYPE"}, {"Level"=3, "Class Only"=FALSE, "Identifier"="RSSCOPE_ATTR_POWER_MODULATION_SOURCE", "Descriptive Name"="Power Modulation Source", "Data Type"=0, "Command"="POW:MOD:SOUR", "Access"=2, "Range Table"="RsScope_rngPowerSource", "Read Callback"="", "Write Callback"="", "Supported Models"="", "Instrument Options"="", "Flags"=0, "Help"="Selects the source for the measurement.\n\nAvailable Repeated Capabilities:\nNone\n\nRemote-control command(s):\nPOWer:MODulation:SOURce"}, {"Level"=3, "Class Only"=FALSE, "Identifier"="RSSCOPE_ATTR_POWER_MODULATION_SCALING", "Descriptive Name"="Power Modulation Scaling", "Data Type"=0, "Command"="POW:MOD:AUTO", "Access"=2, "Range Table"="RsScope_rngPowerScaling", "Read Callback"="", "Write Callback"="", "Supported Models"="", "Instrument Options"="", "Flags"=0, "Help"="Selects the scaling for the display of the results.\n\nAvailable Repeated Capabilities:\nNone\n\nRemote-control command(s):\nPOWer:MODulation:AUTO"}, {"Level"=3, "Class Only"=FALSE, "Identifier"="RSSCOPE_ATTR_POWER_MODULATION_HISTOGRAM", "Descriptive Name"="Power Modulation Histogram", "Data Type"=3, "Command"="POW:MOD:DHIS", "Access"=2, "Range Table"="", "Read Callback"="", "Write Callback"="", "Supported Models"="", "Instrument Options"="", "Flags"=0, "Help"="Activates or deactivates the display of a histogram.\n\nNote: Available only for type continuous\n\nAvailable Repeated Capabilities:\nNone\n\nRemote-control command(s):\nPOWer:MODulation:DHIStogram"}, {"Level"=3, "Class Only"=FALSE, "Identifier"="RSSCOPE_ATTR_POWER_MODULATION_ADD", "Descriptive Name"="Power Modulation Add To Report", "Data Type"=4, "Command"="POW:MOD:REP:ADD", "Access"=1, "Range Table"="", "Read Callback"="", "Write Callback"="", "Supported Models"="", "Instrument Options"="", "Flags"=0, "Help"="Adds the result to the report list.\n\nAvailable Repeated Capabilities:\nNone\n\nRemote-control command(s):\nPOWer:MODulation:REPort:ADD"}, {"Level"=3, "Class Only"=TRUE, "Identifier"="", "Descriptive Name"="Results", "Data Type"=0, "Command"="", "Access"=0, "Range Table"="", "Read Callback"="", "Write Callback"="", "Supported Models"="", "Instrument Options"="", "Flags"=0, "Help"="Results of the modulation measurement."}, {"Level"=2, "Class Only"=TRUE, "Identifier"="", "Descriptive Name"="Dynamic On Resistance", "Data Type"=0, "Command"="", "Access"=0, "Range Table"="", "Read Callback"="", "Write Callback"="", "Supported Models"="", "Instrument Options"="", "Flags"=0, "Help"="Dynamic On Resistance Measurement."}, {"Level"=3, "Class Only"=FALSE, "Identifier"="RSSCOPE_ATTR_START_POWER_DYNAMIC_ON_RESISTANCE_MEASUREMENT", "Descriptive Name"="Start Power Dynamic On Resistance Measurement", "Data Type"=4, "Command"="POW:DONR:EXEC", "Access"=1, "Range Table"="", "Read Callback"="", "Write Callback"="", 
